vi "Oscilloscope.vi"(3 "error in (no error)":errorcluster, 6 "Data In":string) -> (0 "error out (no error)":errorcluster, 2 "Data out":string)   [LabVIEW 2011]
doc: "Oscilloscope\n\nThis is the top vi for communication with the oscilloscope. It contain both a setup and a fetch data command."
uses:
  Server_Globals.vi
panel:
  # "Initialization"
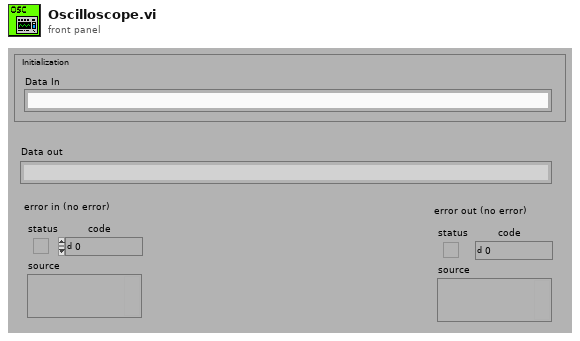
[diagram p1: front panel]
types:
  T1 = cluster{"I/O Settings":u64[], "Instrument Handle":cluster{"5402":refnum<k15>, " 5112":refnum<k15>, "4072":refnum<k15>, "USB":refnum<visa-resource-name>, "4110":refnum<k15>}, "Logfile":refnum<file>, "Log Level":i8, "Clear":i32[], "OS Set":cluster{"instrument handle out":refnum<k15>, "remaining string":string, "Settings":cluster{"Horizontal Conf.":cluster{"Min. Sample rate":dbl, "Reference position":dbl, "Record Length":i16}, "Channel A":cluster{"Enable":bool, "Vertical coupling":dbl, "Vertical range":dbl, "Vertical offset":dbl, "Probe attenuation":dbl}, "Channel B":cluster{"Enable":bool, "Vertical coupling":dbl, "Vertical range":dbl, "Vertical offset":dbl, "Probe attenuation":dbl}, "Trigger":cluster{"Source":enum8{"channel 1", "channel 2", "Imediate", "External trigger"}, "Slope":enum8{"Positive", "Negative"}, "Coupling":enum8{"AC", "DC"}, "Level":dbl, "Holdoff":dbl, "Delay":dbl, " Timeout":dbl, " Mode":enum8{"Normal", "Auto", "Auto Level"}}, "Measurements":cluster{"Measurement 1, Channel":enum8{"Channel 1", "Channel 2", "Channel 3", "Channel 4"}, "Measurement 1, Selection":u16, "Measurement 2, Channel":enum8{"Channel 1", "Channel 2", "Channel 3", "Channel 4"}, "Measurement 2,  Selection":u16, "Measurement 3, Channel":enum8{"Channel 1", "Channel 2", "Channel 3", "Channel 4"}, "Measurement 3, Selection 3":u16}}}, "DC Power Supply":cluster{"0":refnum<k15>, "1":refnum<k15>, "2":refnum<k15>, "3":refnum<k15>, "4":refnum<k15>}, "USB Interface":cluster{"0":refnum<visa-resource-name>, "1":refnum<visa-resource-name>, "2":refnum<visa-resource-name>, "3":refnum<visa-resource-name>, "4":refnum<visa-resource-name>}, "Function Generator":cluster{"0":refnum<k15>, "1":refnum<k15>, "2":refnum<k15>, "3":refnum<k15>, "4":refnum<k15>}, "Digital Multimeter":cluster{"0":refnum<k15>, "1":refnum<k15>, "2":refnum<k15>, "3":refnum<k15>, "4":refnum<k15>}, "Digital Osciliscope":cluster{"0":refnum<k15>, "1":refnum<k15>, "2":refnum<k15>, "3":refnum<k15>, "4":refnum<k15>}, "To M Server":string, "Adres":string[][], "Matrix version":string, "MD5":string, "Digital Multimeter Card 2":cluster{"0":string, "1":string, "2":string, "3":string, "4":string}}
  T2 = cluster{"0":refnum<k15>, "1":refnum<k15>, "2":refnum<k15>, "3":refnum<k15>, "4":refnum<k15>}
  T3 = cluster{"instrument handle out":refnum<k15>, "remaining string":string, "Settings":cluster{"Horizontal Conf.":cluster{"Min. Sample rate":dbl, "Reference position":dbl, "Record Length":i16}, "Channel A":cluster{"Enable":bool, "Vertical coupling":dbl, "Vertical range":dbl, "Vertical offset":dbl, "Probe attenuation":dbl}, "Channel B":cluster{"Enable":bool, "Vertical coupling":dbl, "Vertical range":dbl, "Vertical offset":dbl, "Probe attenuation":dbl}, "Trigger":cluster{"Source":enum8{"channel 1", "channel 2", "Imediate", "External trigger"}, "Slope":enum8{"Positive", "Negative"}, "Coupling":enum8{"AC", "DC"}, "Level":dbl, "Holdoff":dbl, "Delay":dbl, " Timeout":dbl, " Mode":enum8{"Normal", "Auto", "Auto Level"}}, "Measurements":cluster{"Measurement 1, Channel":enum8{"Channel 1", "Channel 2", "Channel 3", "Channel 4"}, "Measurement 1, Selection":u16, "Measurement 2, Channel":enum8{"Channel 1", "Channel 2", "Channel 3", "Channel 4"}, "Measurement 2,  Selection":u16, "Measurement 3, Channel":enum8{"Channel 1", "Channel 2", "Channel 3", "Channel 4"}, "Measurement 3, Selection 3":u16}}}
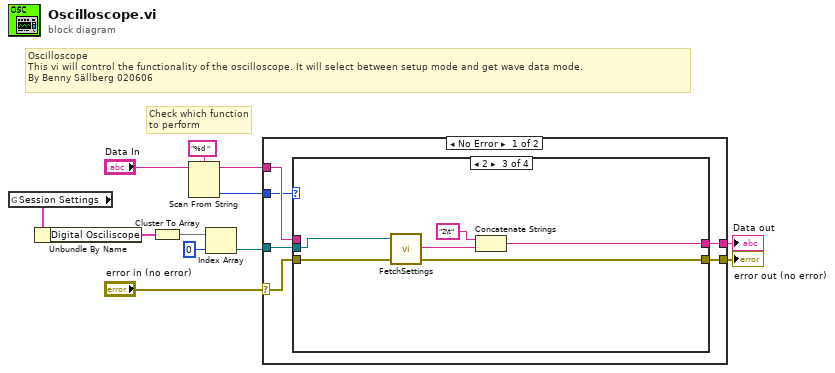
[diagram p0: block diagram]
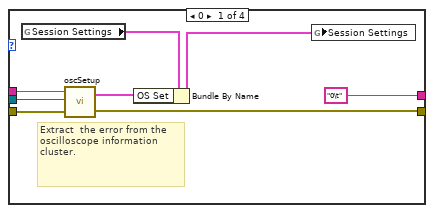
[diagram p2: hidden frame]
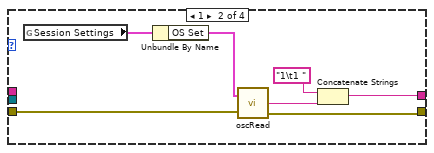
[diagram p3: hidden frame]
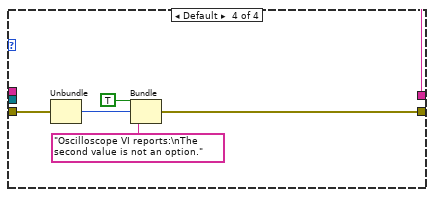
[diagram p4: hidden frame]
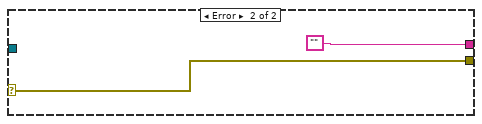
[diagram p5: hidden frame]
diagram:
  # "Check which function\nto perform"
  # "Oscilloscope\nThis vi will control the functionality of the oscilloscope. It will select between setup mode and get wave data mode.\nBy Benny Sällberg 020606"
  n1 = global read "Server_Globals.vi" "Session Settings"() -> (w5:T1)
  n2 = Unbundle By Name(w5) -> ("Digital Osciliscope"=w4:T2)
  n3 = Cluster To Array(cluster=w4) -> (array=w3:refnum<k15>[])
  n4 = Scan From String(format string="%d ", input string="Data In") -> (remaining string=w10:string, output 1=w9:i32)  [unwired: 3 in, 2 out]
  n5 = Index Array(array=w3, index=0) -> (element=w1:refnum<k15>)
  n6 = case shown="No Error" "error in (no error)" {
    selector: "error in (no error)" -> [w15 w47]
    tunnel: [w18 w47] -> w8
    tunnel: w10 -> [w17 _]
    tunnel: w9 -> [w16 _]
    tunnel: w1 -> [w14 _]
    tunnel: [w13 ""] -> w6
    frame No Error {
      n7 = case shown="2" w16 {
        tunnel: [w21 w28 w37 w40] -> w18
        tunnel: w17 -> [w26 _ _ _]
        tunnel: ["0\t" w32 w36 ""] -> w13
        tunnel: w15 -> [w22 w33 w38 w41]
        tunnel: w14 -> [w19 _ w39 _]
        frame 0 {
          (unwired) ""
          # "Extract  the error from the oscilloscope information cluster."
          # "Setup Oscilloscope Function"
          n8 = global read "Server_Globals.vi" "Session Settings"() -> (w23:T1)
          n9 = call "oscSetup.vi"("error in"=w22, "resource name 5112"=w19, "Oscilloscope Setting Information String"=w26) -> ("error out"=w21:errorcluster, "output cluster"=w20:T3)
          n10 = Bundle By Name(cluster=w23, "OS Set"=w20) -> (w24:T1)
          n11 = global write "Server_Globals.vi" "Session Settings"(w24) -> ()
        }
        frame 1 {
          # "Fetch Oscilloscope Data Function"
          n12 = global read "Server_Globals.vi" "Session Settings"() -> (w30:T1)
          n13 = Unbundle By Name(w30) -> ("OS Set"=w29:T3)
          n14 = call "oscRead.vi"("input cluster"=w29, "error in"=w33) -> ("Output String"=w27:string, "error out (no error)"=w28:errorcluster)  [unwired: 1 out]
          n15 = Concatenate Strings("1\t1 ", w27) -> (w32:string)
        }
        frame 2 {
          n16 = call "FetchSettings.vi"("error in (no error)"=w38, "resource name 5112"=w39) -> ("error out (no error)"=w37:errorcluster, "DataOut"=w35:string)  [unwired: 2 in]
          n17 = Concatenate Strings("2\t", w35) -> (w36:string)
        }
        frame Default {
          n18 = Unbundle(w41) -> ("code"=w42:i32)  [unwired: 2 out]
          n19 = Bundle("status"=TRUE, "code"=w42, "Oscilloscope VI reports:\nThe second value is not an option.") -> (w40:cluster{"status":bool, "code":i32, string})  [unwired: 1 in]
        }
      }
    }
    frame Error {
    }
  }
  "error out (no error)" <- w8
  "Data out" <- w6
